vi "User Defined Type Server.vi"() -> ()   [LabVIEW 2020]
uses:
  source/Server/Server/Server.lvclass
  source/PV Data/PV Data.lvlib
  source/Server/Server/Fetch - Variant.vi
  source/Server/Server/Add PV - Variant.vi
  source/Server/Server/Post - Variant.vi
  source/PV Data/EPICS Time Stamp.ctl
  Custom Structure.ctl
panel:
  in  "Cluster":T1={"fieldA"=123, "fieldB"="Hello!", "fieldC"={"fieldC1"=TRUE, "fieldC2"=98.765}, "timeStamp"={"secondsPastEpoch"=0, "nanoseconds"=0, "userTag"=0}}
  in  "PV name":string="DEV:NDLT2043:STRUCT"
  in  "stop":bool
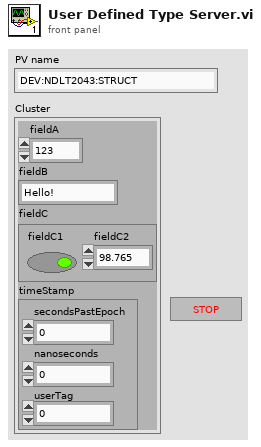
[diagram p1: front panel]
types:
  T1 = typedef "Custom Structure.ctl" = cluster{"fieldA":i32, "fieldB":string, "fieldC":cluster{"fieldC1":bool, "fieldC2":dbl}, "timeStamp":T2}
  T2 = typedef "PV Access.lvlib/PV Data.lvlib/EPICS Time Stamp.ctl" = cluster{"secondsPastEpoch":i64, "nanoseconds":i32, "userTag":i32}
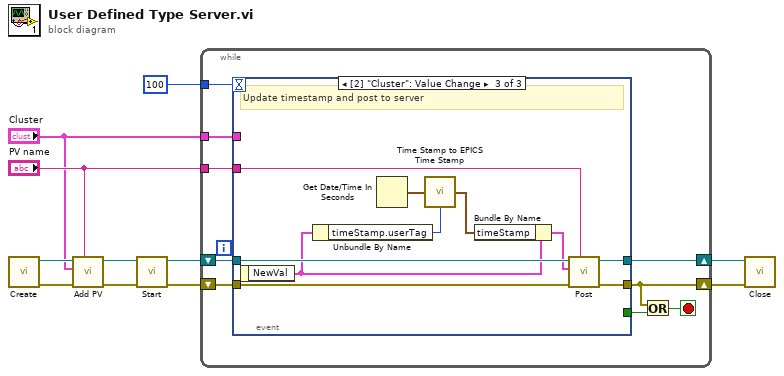
[diagram p0: block diagram]
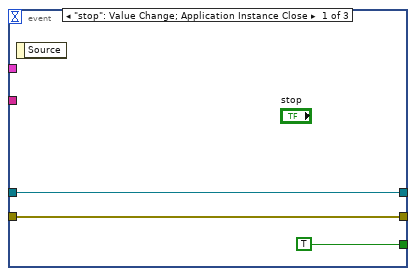
[diagram p2: hidden frame]
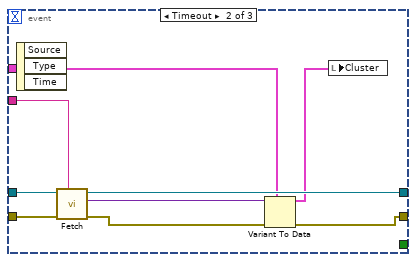
[diagram p3: hidden frame]
diagram:
  n1 = call "Create.vi"() -> ("error out"=w1:errorcluster, "Server out"=w8:refnum<class "Server.lvclass">)  [unwired: 10 in]
  n2 = call-poly "Add PV.vi"("PV name"="PV name", "error in (no error)"=w1, "initial value"="Cluster", "Server in"=w8) -> ("error out"=w6:errorcluster, "Server out"=w5:refnum<class "Server.lvclass">)  [unwired: 5 in, 1 out]
  n3 = call-dynamic "Start.vi"("error in (no error)"=w6, "Server in"=w5) -> ("error out"=w3:errorcluster, "Server out"=w4:refnum<class "Server.lvclass">)  [unwired: 8 in]
  n4 = while {
    tunnel: "PV name" -> [w19]
    shift-right: [w17] -> w9
    shift-left: w4 -> [w18]
    shift-right: [w14] -> w10
    shift-left: w3 -> [w20]
    tunnel: 100 ("Numeric") -> [w13]
    tunnel: "Cluster" -> [w12]
    stop <- w15 stop-if-true
    n5 = event shown="[2] \"Cluster\": Value Change" {
      selector: _ -> [_ _ _]
      dyn-events: _ -> [_ _ _]
      timeout: w13 -> [_ _ _]
      tunnel: w20 -> [w22 w32 w38]
      tunnel: w19 -> [_ w30 w41]
      tunnel: w18 -> [w21 w31 w40]
      tunnel: [w22 w26 w42] -> w14
      tunnel: [w21 w29 w39] -> w17
      tunnel: [TRUE _ _] -> w16
      tunnel: w12 -> [_ w24 _]
      event "stop": Value Change; Application Instance Close {
        n6 = event-data() -> ()  [unwired: 1 in, 1 out]
      }
      event Timeout {
        n7 = event-data() -> ()  [unwired: 1 in, 3 out]
        n8 = call-poly "Fetch.vi"("PV name"=w30, "error in"=w32, "Server in"=w31) -> ("error out"=w27:errorcluster, "value"=w25:variant, "Server out"=w29:refnum<class "Server.lvclass">)  [unwired: 5 in, 1 out]
        n9 = Variant To Data(error in=w27, type=w24, Variant=w25) -> (data=w28:T1, error out=w26:errorcluster)
        n10 = local write "Cluster"(w28) -> ()
      }
      event Value Change {
        # "Update timestamp and post to server"
        n11 = event-data() -> ("NewVal"=w36:T1)  [unwired: 1 in]
        n12 = Unbundle By Name(w36) -> ("timeStamp.userTag"=w35:i32)
        n13 = Get Date/Time In Seconds() -> (seconds since 1Jan1904=w37:timestamp)
        n14 = call "Time Stamp to EPICS Time Stamp.vi"("time stamp"=w37, "user tag"=w35) -> ("EPICS time stamp"=w34:T2)
        n15 = Bundle By Name(cluster=w36, "timeStamp"=w34) -> (w33:T1)
        n16 = call-poly "Post.vi"("PV name"=w41, "error in (no error)"=w38, "value"=w33, "Server in"=w40) -> ("error out"=w42:errorcluster, "Server out"=w39:refnum<class "Server.lvclass">)  [unwired: 6 in]
      }
    }
    n17 = Or(x=w14, y=w16) -> (x .or. y?=w15:bool)
  }
  n18 = call-dynamic "Close.vi"("error in"=w10, "Server in"=w9) -> ()  [unwired: 9 in, 1 out]
